vi "TxT2DATA.vi"(10 "Text Data":string, 11 "Text_Format":T1) -> (3 "Data":i32[](array[numeric]))   [LabVIEW 2020, in "Text File.lvclass"]
uses:
  Text File.lvclass
  Text File.lvclass/Text File.ctl
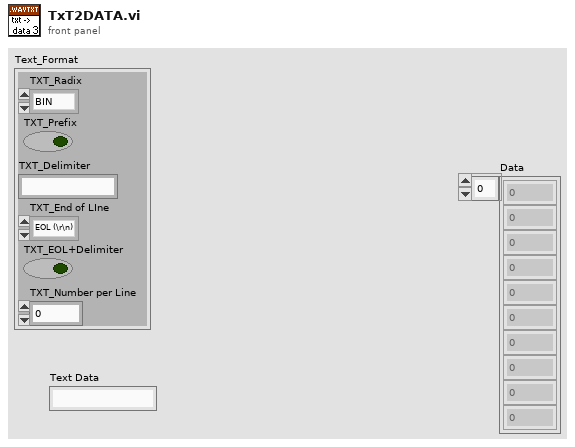
[diagram p1: front panel]
types:
  T1 = cluster{"TXT_Radix":enum16{"BIN", "DEC", "HEX"}, "TXT_Prefix":bool, "TXT_Delimiter":string, "TXT_End of LIne":enum16{"EOL (\\r\\n)", "LF (\\n)"}, "TXT_EOL+Delimiter":bool, "TXT_Number per Line":i32}
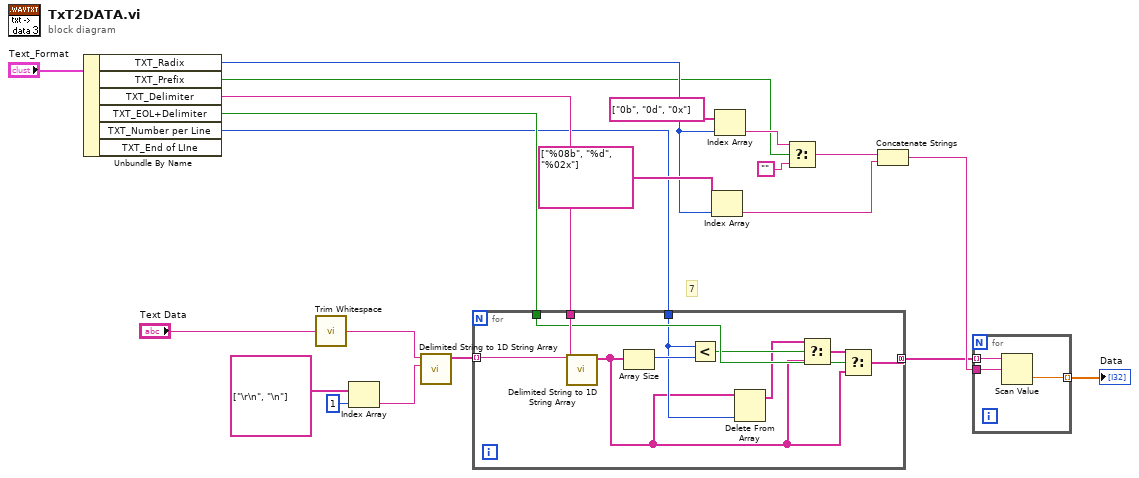
[diagram p0: block diagram]
diagram:
  # "7"
  n1 = Unbundle By Name("Text_Format") -> ("TXT_Radix"=w6:enum16{"BIN", "DEC", "HEX"}, "TXT_Prefix"=w5:bool, "TXT_Delimiter"=w4:string, "TXT_EOL+Delimiter"=w3:bool, "TXT_Number per Line"=w2:i32)  [unwired: 1 out]
  n2 = call <vilib>:"Trim Whitespace.vi"("string"="Text Data") -> ("trimmed string"=w13:string)  [unwired: 1 in]
  n3 = Index Array(array=string[] ["\r\n", "\n"], index=1 ("인덱스")) -> (element=w11:string)
  n4 = call <vilib>:"Delimited String to 1D String Array.vi"("delimiter"=w11, "delimited string"=w13) -> ("string array"=w10:string[])  [unwired: 9 in]
  n5 = for {
    tunnel: w10 -> [w30] mode=indexing
    tunnel: [w29] -> w9 mode=concatenating
    tunnel: w4 -> [w31]
    tunnel: w3 -> [w27]
    tunnel: w2 -> [w25]
    n6 = call <vilib>:"Delimited String to 1D String Array.vi"("delimiter"=w31, "delimited string"=w30) -> ("string array"=w22:string[])  [unwired: 9 in]
    n7 = Array Size(array=w22) -> (size(s)=w28:i32)
    n8 = Less?(x=w25, y=w28) -> (x < y?=w26:bool)
    n9 = Delete From Array(array=w22, index=w25) -> (array with subset deleted=w23:string[])  [unwired: 1 in, 1 out]
    n10 = Select(t=w23, s=w26, f=w22) -> (s? t:f=w24:string[])
    n11 = Select(t=w24, s=w27, f=w22) -> (s? t:f=w29:string[])
  }
  n12 = Index Array(array=string[] ["%08b", "%d", "%02x"], index=w6) -> (element=w19:string)
  n13 = Index Array(array=string[] ["0b", "0d", "0x"], index=w6) -> (element=w16:string)
  n14 = Select(t=w16, s=w5, f="") -> (s? t:f=w14:string)
  n15 = Concatenate Strings(w14, w19) -> (w18:string)
  n16 = for {
    tunnel: w18 -> [w34]
    tunnel: [w33] -> w17 mode=indexing
    tunnel: w9 -> [w32] mode=indexing
    n17 = Scan Value(string=w32, format string=w34) -> (value=w33:dbl)  [unwired: 1 in, 1 out]
  }
  "Data" <- w17
